vi "FalseColorIntensityAxis.vi"(7 "Inverse":bool, 9 "Offset":dbl, 10 "ViewColor":bool, 11 "Scale":dbl=1.0) -> (3 "ZScaleMarkerVals":cluster{dbl, "Color Box":u32}[](array[cluster]))   [LabVIEW 2023]
doc: "This convenience VI creates the colour markers for an intensity graph in rainbow style (blue to red).\nUse this VI to rescale the Z-axis in an IntensityImage.\n\ninfo@becker-hickl.com"
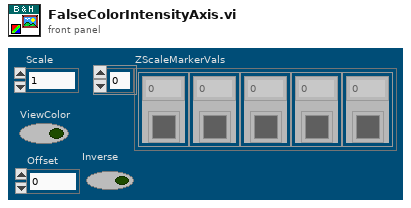
[diagram p1: front panel]
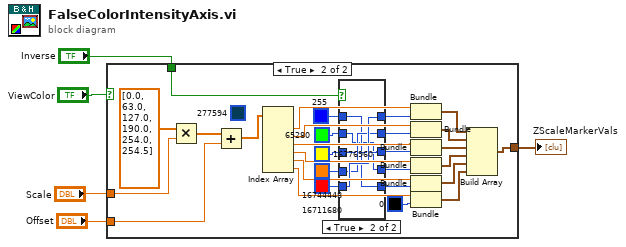
[diagram p0: block diagram]
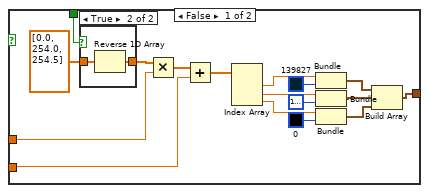
[diagram p2: hidden frame]
diagram:
  n1 = case shown="True" "ViewColor" {
    tunnel: [w16 w45] -> w2
    tunnel: "Scale" -> [w12 w44]
    tunnel: "Offset" -> [w9 w42]
    tunnel: "Inverse" -> [w6 w41]
    frame False {
      n2 = case shown="True" w6 {
        tunnel: dbl[] [0.0, 254.0, 254.5] -> [w23 w25]
        tunnel: [w23 w24] -> w7
        frame False {
        }
        frame True {
          n3 = Reverse 1D Array(array=w25) -> (reversed array=w24:dbl[])
        }
      }
      n4 = Multiply(x=w7, y=w12) -> (x*y=w11:dbl[])
      n5 = Add(x=w11, y=w9) -> (x+y=w10:dbl[])
      n6 = Index Array(array=w10) -> (element #1=w15:dbl, element #2=w14:dbl, element #3=w13:dbl)  [unwired: 3 in]
      n7 = Bundle(w15, "Color Box"=u32 139827) -> (w22:cluster{dbl, "Color Box":u32})  [unwired: 1 in]
      n8 = Bundle(w14, "Color Box"=u32 16777225) -> (w21:cluster{dbl, "Color Box":u32})  [unwired: 1 in]
      n9 = Bundle(w13, "Color Box"=u32 0) -> (w20:cluster{dbl, "Color Box":u32})  [unwired: 1 in]
      n10 = Build Array(w22, w21, w20) -> (w16:cluster{dbl, "Color Box":u32}[])
    }
    frame True {
      (unwired) u32 277594 ("Color Box")
      n11 = Multiply(x=dbl[] [0.0, 63.0, 127.0, 190.0, 254.0, 254.5], y=w44) -> (x*y=w46:dbl[])
      n12 = Add(x=w46, y=w42) -> (x+y=w43:dbl[])
      n13 = Index Array(array=w43) -> (element #1=w49:dbl, element #2=w48:dbl, element #3=w47:dbl, element #4=w53:dbl, element #5=w27:dbl, element #6=w30:dbl)  [unwired: 6 in]
      n14 = case shown="True" w41 {
        tunnel: u32 255 ("Color Box") -> [w60 w62]
        tunnel: [w60 w65] -> w39
        tunnel: u32 65280 ("Color Box") -> [w59 w61]
        tunnel: [w59 w64] -> w37
        tunnel: u32 16776960 ("Color Box") -> [w58 w63]
        tunnel: [w58 w63] -> w35
        tunnel: u32 16711680 ("Color Box") -> [w57 w65]
        tunnel: [w56 w61] -> w33
        tunnel: [w57 w62] -> w29
        tunnel: u32 16744448 ("Color Box") -> [w56 w64]
        frame False {
        }
        frame True {
        }
      }
      n15 = Bundle(w49, "Color Box"=w39) -> (w52:cluster{dbl, "Color Box":u32})  [unwired: 1 in]
      n16 = Bundle(w48, "Color Box"=w37) -> (w51:cluster{dbl, "Color Box":u32})  [unwired: 1 in]
      n17 = Bundle(w47, "Color Box"=w35) -> (w50:cluster{dbl, "Color Box":u32})  [unwired: 1 in]
      n18 = Bundle(w53, "Color Box"=w33) -> (w55:cluster{dbl, "Color Box":u32})  [unwired: 1 in]
      n19 = Bundle(w27, "Color Box"=w29) -> (w31:cluster{dbl, "Color Box":u32})  [unwired: 1 in]
      n20 = Bundle(w30, "Color Box"=u32 0) -> (w32:cluster{dbl, "Color Box":u32})  [unwired: 1 in]
      n21 = Build Array(w52, w51, w50, w55, w31, w32) -> (w45:cluster{dbl, "Color Box":u32}[])
    }
  }
  "ZScaleMarkerVals" <- w2
